vi "BuildFCPPacket.vi"(6 "Data":u32[](array[numeric]), 8 "Data Length (in Bytes)":u32, 9 "SequenceNumber":u32, 10 "Channel":u32, 11 "Command":u32) -> (3 "FCP Packet":u32[](array[numeric]))   [LabVIEW 2009]
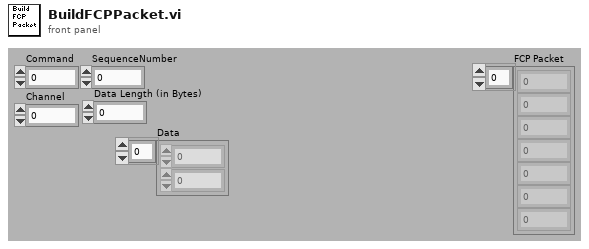
[diagram p1: front panel]
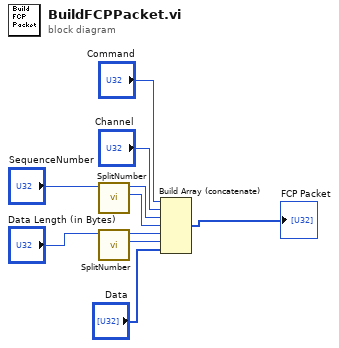
[diagram p0: block diagram]
diagram:
  n1 = call "SplitNumber.vi"("x"="SequenceNumber") -> ("Lower"=w7:u32, "Upper"=w8:u32)  [unwired: 9 in]
  n2 = call "SplitNumber.vi"("x"="Data Length (in Bytes)") -> ("Lower"=w5:u32, "Upper"=w6:u32)  [unwired: 9 in]
  n3 = Build Array (concatenate)("Command", "Channel", w8, w7, w6, w5, "Data") -> (→"FCP Packet":u32[])
